vi "Read output range.vi"(8 "error in (no error)":errorcluster, 11 "PID in":refnum<class "PID.lvclass">) -> (0 "error out":errorcluster, 2 "output range":cluster{"output high":dbl, "output low":dbl}={"output high"=100.0, "output low"=-100.0} {"output low" format="%.2f"; "output high" format="%.2f"}, 3 "PID out":refnum<class "PID.lvclass">)   [LabVIEW 2024, in "PID.lvlib" / "PID.lvclass"]
uses:
  PID.lvclass
  PID.lvclass/PID.ctl
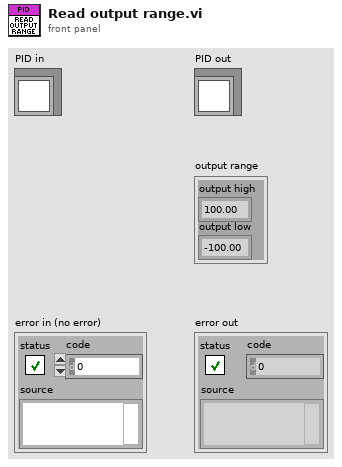
[diagram p1: front panel]
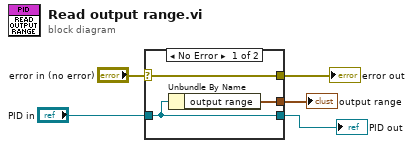
[diagram p0: block diagram]
diagram:
  n1 = case shown="No Error" "error in (no error)" {
    selector: "error in (no error)" -> [w8 w9]
    tunnel: [w8 w9] -> w4
    tunnel: [w7 w10] -> w2
    tunnel: "PID in" -> [w7 w10]
    tunnel: [w6 _] -> w1
    frame No Error {
      n2 = Unbundle By Name(w7) -> ("output range"=w6:cluster{"output high":dbl, "output low":dbl})
    }
    frame Error {
    }
  }
  "error out" <- w4
  "PID out" <- w2
  "output range" <- w1
